vi "FPGA - Calculate Delay Addresses.vi"(10 "Delay_ticks":u32, 11 "index":i32) -> (2 "Read Address":u32, 3 "Write Address":u32)   [LabVIEW 2014]
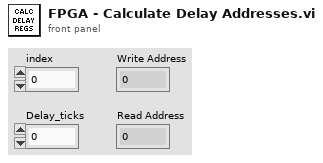
[diagram p1: front panel]
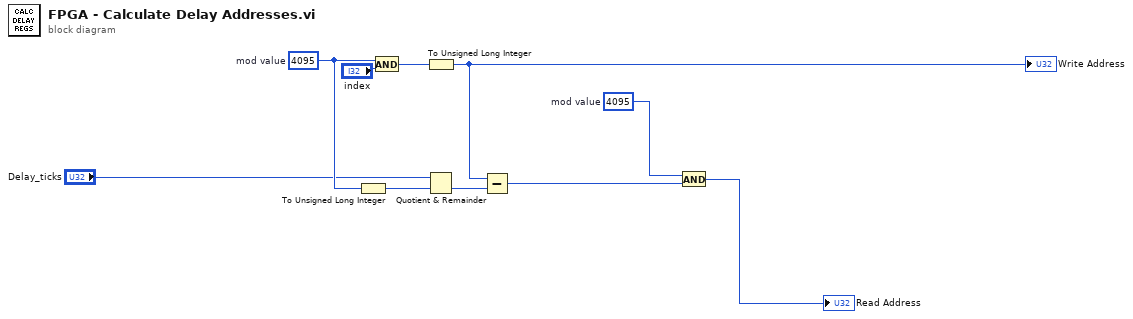
[diagram p0: block diagram]
diagram:
  w8 = u32 4095  # mod value
  w4 = 4095  # mod value
  n1 = To Unsigned Long Integer(number=w4) -> (unsigned 32bit integer=w5:u32)
  n2 = And(x=w4, y="index") -> (x .and. y?=w2:i32)
  n3 = To Unsigned Long Integer(number=w2) -> (unsigned 32bit integer=w9:u32)
  "Write Address" <- w9
  n4 = Quotient & Remainder(x="Delay_ticks", y=w5) -> (floor(x/y)=w6:u32)  [unwired: 1 out]
  n5 = Subtract(x=w9, y=w6) -> (x-y=w7:u32)
  n6 = And(x=w8, y=w7) -> (x .and. y?=→"Read Address":u32)
